vi "p1.vi"() -> ()   [LabVIEW 2021, in "d25.lvlib"]
uses:
  d25.lvlib
  AOC/AOC.lvlib
panel:
  out "SNAFU":string
  in  "Example":string="1=-0-2\n12111\n2=0=\n21\n2=01\n111\n20012\n112\n1=-1=\n1-12\n12\n1=\n122"
  in  "Example":bool
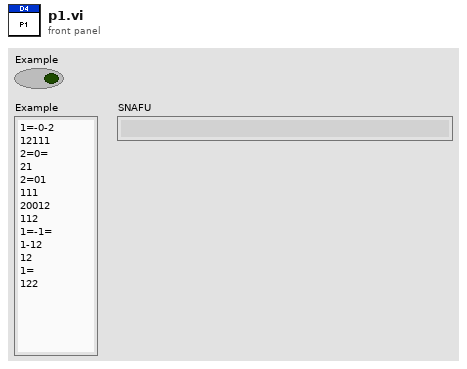
[diagram p1: front panel]
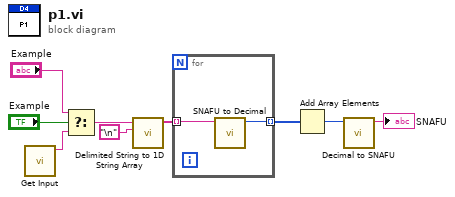
[diagram p0: block diagram]
diagram:
  n1 = call "Get Input.vi"() -> ("Input"=w9:string)  [unwired: 11 in]
  n2 = Select(t="Example", s="Example", f=w9) -> (s? t:f=w8:string)
  n3 = call <vilib>:"Delimited String to 1D String Array.vi"("delimiter"="\n", "delimited string"=w8) -> ("string array"=w4:string[])  [unwired: 9 in]
  n4 = for {
    tunnel: w4 -> [w11] mode=indexing
    tunnel: [w10] -> w3 mode=indexing
    n5 = call "SNAFU to Decimal.vi"("SNAFU"=w11) -> ("Decimal"=w10:i64)  [unwired: 10 in]
  }
  n6 = Add Array Elements(numeric array=w3) -> (sum=w2:i64)
  n7 = call "Decimal to SNAFU.vi"("Decimal"=w2) -> ("SNAFU"=→"SNAFU":string)  [unwired: 10 in]
